vi "SwerveJoystickStrafeScaling.vi"(0 "Raw Joystick X":dbl, 1 "Slew Rate Limit (/s)":dbl=1.0, 5 "Raw Joystick Y":dbl, 7 "Auto Control":bool, 9 "Strafe Deadband":dbl(slide)=0.05 min=0.0 max=0.25 scale=0.0..0.25, 11 "Strafe Scaling":dbl(slide)=2.0 min=1.0 max=4.0 scale=1.0..4.0, 12 "Strafe Maximum":dbl(slide)=0.5 min=0.3 max=1.0 scale=0.3..1.0) -> (4 "In Deadband":bool, 8 "Scaled Joystick X":dbl format="%.2f", 15 "Scaled Joystick Y":dbl format="%.2f")   [LabVIEW 2020]
doc: "Applies a deadband and nonlinear scaling to the strafe axes of a swerve drive. Includes a hook to override the non-linear deadband and scaling when the rotation is under autonomous control. Includes a de-saturation check to handle compounding drive commands from different controllers (e.g. direct driver control + auto targeting)."
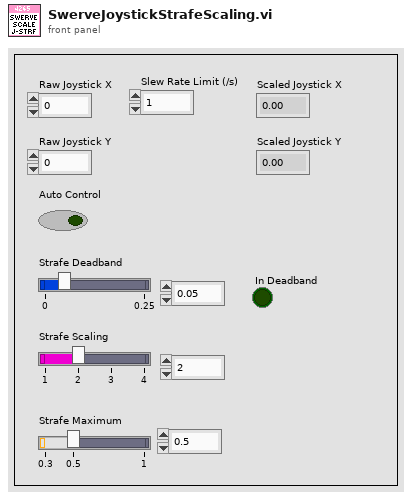
[diagram p1: front panel]
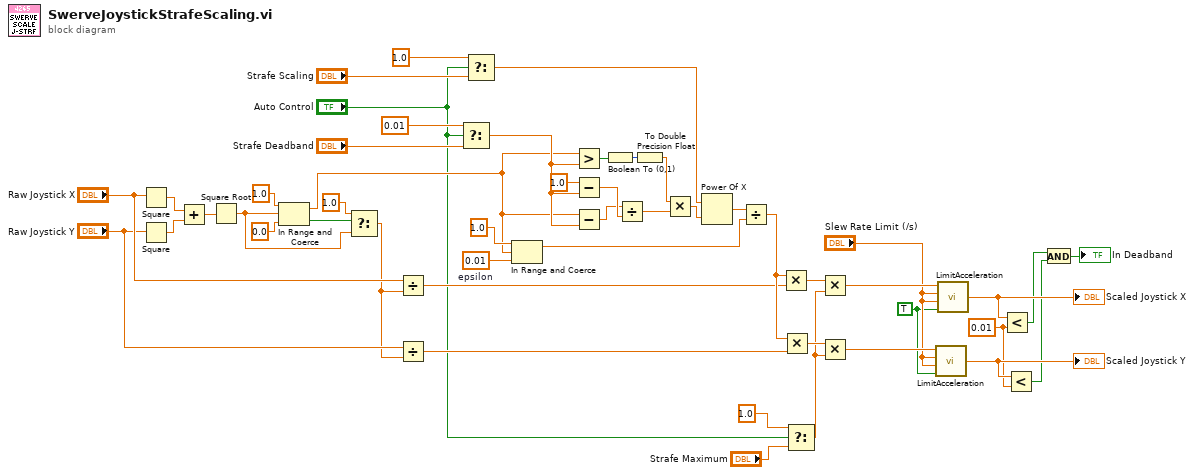
[diagram p0: block diagram]
diagram:
  w4 = 0.01 ("upper limit")
  w11 = TRUE ("Apply Limit")
  w44 = 0.01  # epsilon
  n1 = Square(x="Raw Joystick X") -> (x^2=w41:dbl)
  n2 = Square(x="Raw Joystick Y") -> (x^2=w40:dbl)
  n3 = Add(x=w41, y=w40) -> (x+y=w42:dbl)
  n4 = Square Root(x=w42) -> (sqrt(x)=w23:dbl)
  n5 = In Range and Coerce(upper limit=1.0, x=w23, lower limit=0.0 ("upper limit")) -> (coerced(x)=w17:dbl, In Range?=w25:bool)
  n6 = Select(t=1.0, s=w25, f=w23) -> (s? t:f=w18:dbl)
  n7 = Divide(x="Raw Joystick X", y=w18) -> (x/y=w22:dbl)
  n8 = Divide(x="Raw Joystick Y", y=w18) -> (x/y=w19:dbl)
  n9 = Select(t=0.01, s="Auto Control", f="Strafe Deadband") -> (s? t:f=w28:dbl)
  n10 = Select(t=1.0, s="Auto Control", f="Strafe Scaling") -> (s? t:f=w29:dbl)
  n11 = In Range and Coerce(upper limit=1.0, x=w17, lower limit=w44) -> (coerced(x)=w43:dbl)  [unwired: 1 out]
  n12 = Greater?(x=w17, y=w28) -> (0:w47:bool)
  n13 = Subtract(x=1.0, y=w28) -> (x-y=w38:dbl)
  n14 = Subtract(x=w17, y=w28) -> (x-y=w36:dbl)
  n15 = Boolean To (0,1)(Boolean=w47) -> (0, 1=w34:i16)
  n16 = Divide(x=w36, y=w38) -> (x/y=w39:dbl)
  n17 = To Double Precision Float(number=w34) -> (double precision float=w35:dbl)
  n18 = Multiply(x=w35, y=w39) -> (x*y=w48:dbl)
  n19 = Power Of X(1:w48, 2:w29) -> (0:w49:dbl)
  n20 = Divide(x=w49, y=w43) -> (x/y=w46:dbl)
  n21 = Multiply(x=w46, y=w22) -> (x*y=w15:dbl)
  n22 = Multiply(x=w46, y=w19) -> (x*y=w16:dbl)
  n23 = Select(t=1.0, s="Auto Control", f="Strafe Maximum") -> (s? t:f=w8:dbl)
  n24 = Multiply(x=w15, y=w8) -> (x*y=w14:dbl)
  n25 = Multiply(x=w16, y=w8) -> (x*y=w13:dbl)
  n26 = call "LimitAcceleration.vi"("Apply Limit"=w11, "Decceleration Limit (/s)"="Slew Rate Limit (/s)", "Acceleration Limit (/s)"="Slew Rate Limit (/s)", "Raw Input"=w13) -> ("Output"=w5:dbl)
  "Scaled Joystick Y" <- w5
  n27 = call "LimitAcceleration.vi"("Apply Limit"=w11, "Decceleration Limit (/s)"="Slew Rate Limit (/s)", "Acceleration Limit (/s)"="Slew Rate Limit (/s)", "Raw Input"=w14) -> ("Output"=w6:dbl)
  "Scaled Joystick X" <- w6
  n28 = Less?(x=w6, y=w4) -> (x < y?=w2:bool)
  n29 = Less?(x=w5, y=w4) -> (x < y?=w3:bool)
  n30 = And(x=w2, y=w3) -> (x .and. y?=→"In Deadband":bool)
